vi "Tracking Initialization v2.vi"(5 "Trajectory Cluster":T1, 6 "PID Cluster":T3={"L1 to L4 PID Cluster"={"L1 PID Gains"={"Kp"=0.005, "Kd"=0.5, "Ki"=0.0005}, "L2 PID Gains"={"Kp"=0.01, "Kd"=1.0, "Ki"=0.005}, "L3 PID Gains"={"Kp"=0.05, "Kd"=1.0, "Ki"=0.0005}, "L4 PID Gains"={"Kp"=0.1, "Kd"=0.1, "Ki"=0.0005}}, "Stage PID Cluster"={"Stage Z PID"={"Kp"=0.0005, "Kd"=0.001, "Ki"=0.0}, "Stage Y PID"={"Kp"=0.0003, "Kd"=0.01, "Ki"=0.0}, "Stage X PID"={"Kp"=0.0003, "Kd"=0.01, "Ki"=0.0}}, "OCT Z PID Gains"={"Kp"=0.0003, "Kd"=0.0001, "Ki"=0.01}}, 7 "Offset Home 2 RCM":dbl[](array[numeric])=[0.0, 0.0, 0.0, 0.0], 8 "error in":errorcluster, 10 "Prev Posit Cluster":T4={"Prev L1 to L4 Posit"=[0.0, 0.0, 0.0, 0.0], "Prev Stage Posit"=[6.0, 6.0, 6.0], "Prev OCT Z Posit"=0.0}, 11 "FPGA VI Reference In":refnum<k20>) -> (0 "error out":errorcluster, 2 "Last Posit Cluster":T2={"Last L1 to L4 Posit"=[0.0, 0.0, 0.0, 0.0], "Last Stage Posit"=[6.0, 6.0, 6.0], "Last OCT Z Posit"=0.0}, 3 "FPGA VI Reference Out":refnum<k20>)   [LabVIEW 2016]
uses:
  <vilib>/Platform/TimedLoop/XDataNode/timing_clust.ctl
  <vilib>/Platform/TimedLoop/XDataNode/nitl_modes.ctl
  <vilib>/Platform/TimedLoop/XDataNode/wakeup.ctl
  Global Variables.vi
  <vilib>/platform/TimedLoop/XDataNode/XDataNode.xnode
  <vilib>/Platform/TimedLoop/XDataNode/XDNodeRunTimeDep.lvlib
panel:
  out "In Servo Loop":bool
  out "Indexing Finished?":bool
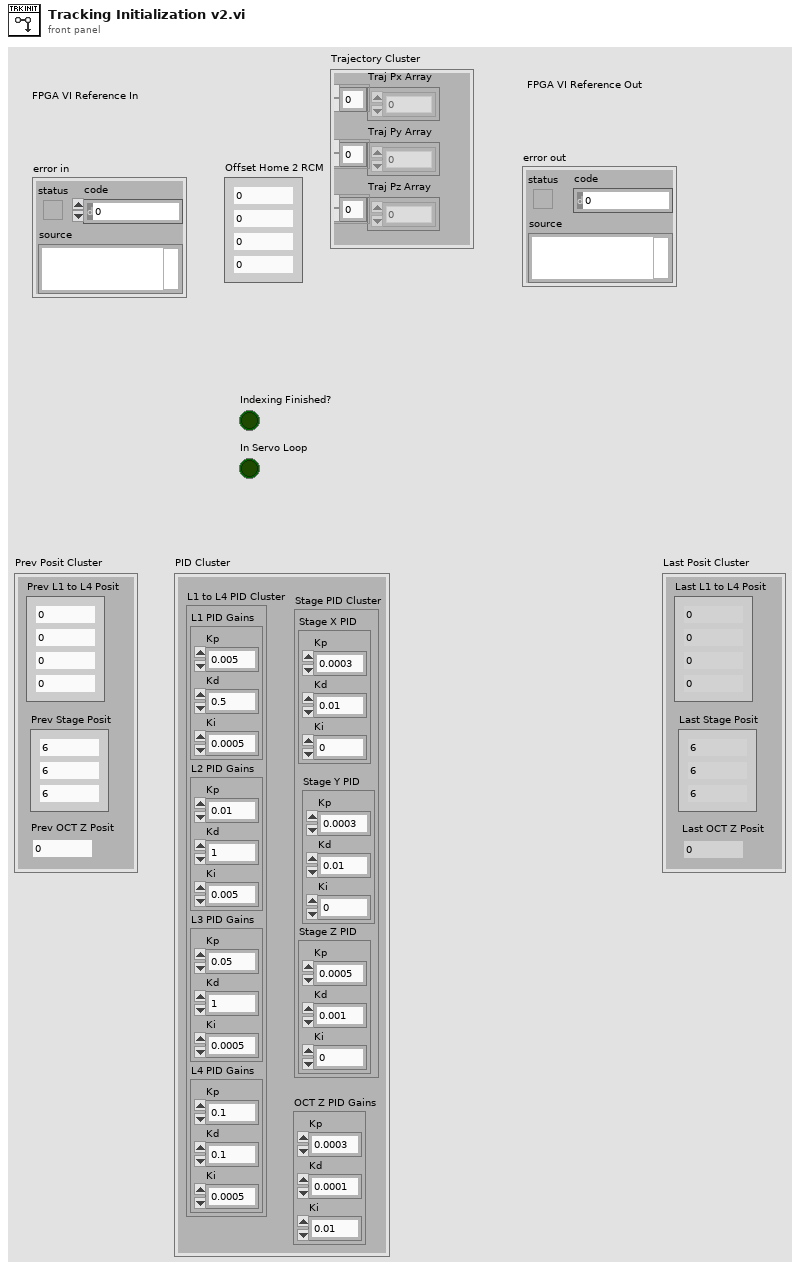
[diagram p1: front panel]
types:
  T1 = cluster{"Traj Px Array":dbl[], "Traj Py Array":dbl[], "Traj Pz Array":dbl[]}
  T2 = cluster{"Last L1 to L4 Posit":dbl[], "Last Stage Posit":dbl[], "Last OCT Z Posit":dbl}
  T3 = cluster{"L1 to L4 PID Cluster":cluster{"L1 PID Gains":cluster{"Kp":dbl, "Kd":dbl, "Ki":dbl}, "L2 PID Gains":cluster{"Kp":dbl, "Kd":dbl, "Ki":dbl}, "L3 PID Gains":cluster{"Kp":dbl, "Kd":dbl, "Ki":dbl}, "L4 PID Gains":cluster{"Kp":dbl, "Kd":dbl, "Ki":dbl}}, "Stage PID Cluster":cluster{"Stage Z PID":cluster{"Kp":dbl, "Kd":dbl, "Ki":dbl}, "Stage Y PID":cluster{"Kp":dbl, "Kd":dbl, "Ki":dbl}, "Stage X PID":cluster{"Kp":dbl, "Kd":dbl, "Ki":dbl}}, "OCT Z PID Gains":cluster{"Kp":dbl, "Kd":dbl, "Ki":dbl}}
  T4 = cluster{"Prev L1 to L4 Posit":dbl[], "Prev Stage Posit":dbl[], "Prev OCT Z Posit":dbl}
  T5 = typedef "XDNodeRunTimeDep.lvlib/timing_clust.ctl" = cluster{"Expected End [f-1]":u64, "Actual End [f-1]":u64, "Finished Late? [f-1]":bool, "Expected End [i-1]":u64, "Actual End [i-1]":u64, "Finished Late? [i-1]":bool, "Expected Start [i]":u64, "Actual Start [i]":u64, "Expected Start [f]":u64, "Actual Start [f]":u64, "Source Name":string, "Structure Name":string, "Period":i64, "Deadline":i64, "Offset":i64, "Start":i64, "Priority":i32, "Timeout":i32, "Mode":T6, "Wakeup Reason":T7, "Error":errorcluster, "Source Type":string, "Secondary Source Type":string, "Global End Time":u64, "Global Start Time":u64, "Frame Duration":u64, "Iteration Duration":u64, "Assigned CPU":i32, "I/O Scan Engine Mode":u32}
  T6 = typedef "XDNodeRunTimeDep.lvlib/nitl_modes.ctl" = enum32{"No Change", "Process missed periods, maintain original phase", "Discard missed periods, maintain original phase", "Process missed periods, ignore original phase", "Discard missed periods, ignore original phase"}
  T7 = typedef "XDNodeRunTimeDep.lvlib/wakeup.ctl" = enum32{"Normal", "Aborted", "Asynchronous wakeup", "Timing source error", "Timed loop error", "Timeout"}
  T8 = cluster{"L1 PID Gains":cluster{"Kp":dbl, "Kd":dbl, "Ki":dbl}, "L2 PID Gains":cluster{"Kp":dbl, "Kd":dbl, "Ki":dbl}, "L3 PID Gains":cluster{"Kp":dbl, "Kd":dbl, "Ki":dbl}, "L4 PID Gains":cluster{"Kp":dbl, "Kd":dbl, "Ki":dbl}}
  T9 = cluster{"Stage Z PID":cluster{"Kp":dbl, "Kd":dbl, "Ki":dbl}, "Stage Y PID":cluster{"Kp":dbl, "Kd":dbl, "Ki":dbl}, "Stage X PID":cluster{"Kp":dbl, "Kd":dbl, "Ki":dbl}}
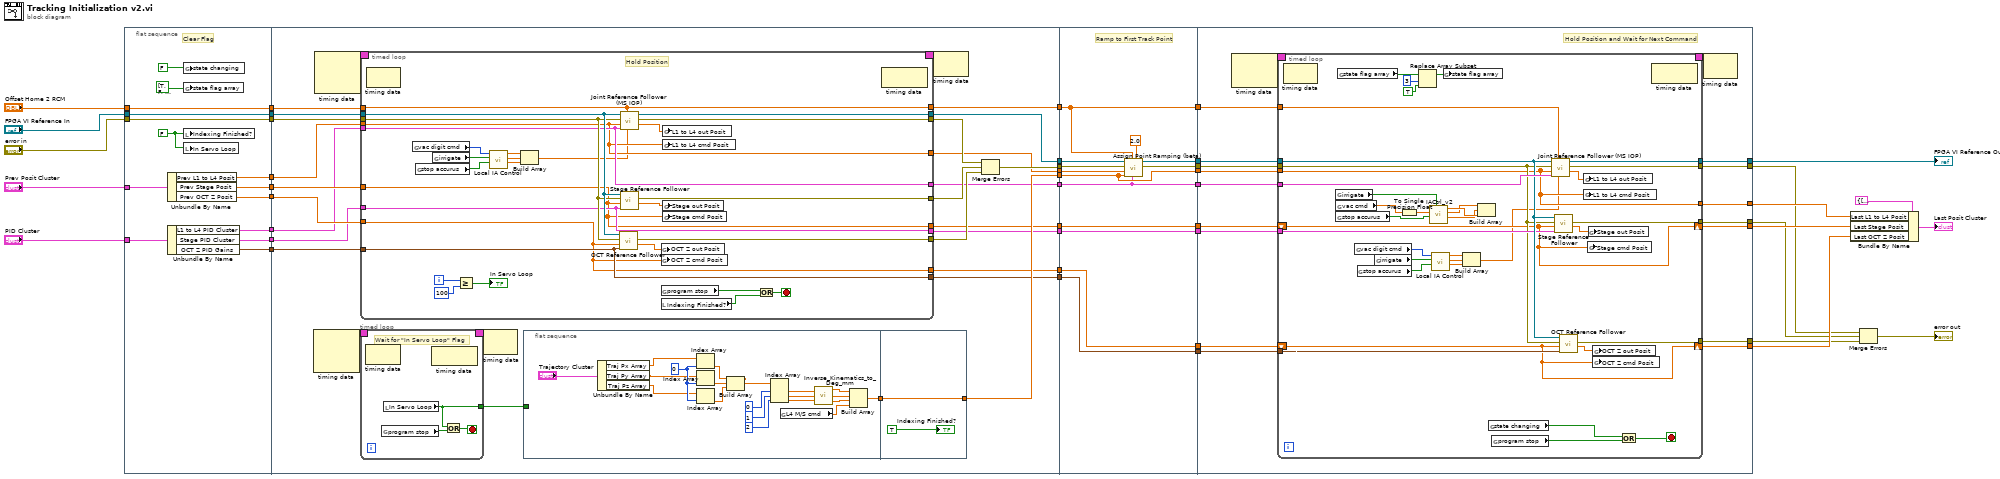
[diagram p0: block diagram]
diagram:
  n1 = flat-sequence {
    tunnel: [w55] -> w21
    tunnel: "FPGA VI Reference In" -> [w55]
    tunnel: "error in" -> [w54]
    tunnel: [w54] -> w19
    tunnel: [w49] -> w17
    tunnel: "PID Cluster" -> [w48]
    tunnel: "Offset Home 2 RCM" -> [w53]
    tunnel: [w53] -> w15
    tunnel: "Prev Posit Cluster" -> [w52]
    tunnel: [w51] -> w12
    tunnel: [w50] -> w10
    tunnel: [w47] -> w8
    tunnel: [w46] -> w7
    tunnel: [w45] -> w6
    tunnel: w21 -> [w82]
    tunnel: [w76] -> w20
    tunnel: w19 -> [w81]
    tunnel: [w72] -> w18
    tunnel: w17 -> [w80]
    tunnel: [w71] -> w16
    tunnel: w15 -> [w83]
    tunnel: [w77] -> w14
    tunnel: [w70] -> w13
    tunnel: w12 -> [w79]
    tunnel: [w68] -> w11
    tunnel: w10 -> [w78]
    tunnel: [w69] -> w9
    tunnel: w8 -> [w67]
    tunnel: w7 -> [w66]
    tunnel: w6 -> [w65]
    tunnel: [w64] -> w5
    tunnel: [w63] -> w3
    tunnel: [w62] -> w1
    tunnel: w20 -> [w160]
    tunnel: w18 -> [w159]
    tunnel: w16 -> [w157]
    tunnel: w14 -> [w154]
    tunnel: w13 -> [w153]
    tunnel: [w156] -> w41
    tunnel: [w153] -> w40
    tunnel: [w155] -> w39
    tunnel: [w154] -> w38
    tunnel: [w150] -> w35
    tunnel: [w148] -> w34
    tunnel: w11 -> [w152]
    tunnel: [w152] -> w22
    tunnel: w9 -> [w149]
    tunnel: w5 -> [w151]
    tunnel: [w151] -> w4
    tunnel: w3 -> [w150]
    tunnel: [w149] -> w2
    tunnel: w1 -> [w148]
    tunnel: [w173] -> w30
    tunnel: [w172] -> w25
    tunnel: w41 -> [w175]
    tunnel: w40 -> [w162]
    tunnel: w39 -> [w176]
    tunnel: w38 -> [w163]
    tunnel: [w171] -> w36
    tunnel: [w170] -> w37
    tunnel: w35 -> [w169]
    tunnel: w34 -> [w168]
    tunnel: [w167] -> w31
    tunnel: [w166] -> w24
    tunnel: [w165] -> w23
    tunnel: w22 -> [w164]
    tunnel: w4 -> [w174]
    tunnel: w2 -> [w161]
    frame #0 {
      w44 = FALSE ("Indexing Finished?")
      # "Clear Flag"
      n2 = Unbundle By Name(w52) -> ("Prev L1 to L4 Posit"=w49:dbl[], "Prev Stage Posit"=w51:dbl[], "Prev OCT Z Posit"=w50:dbl)
      n3 = Unbundle By Name(w48) -> ("L1 to L4 PID Cluster"=w47:T8, "Stage PID Cluster"=w46:T9, "OCT Z PID Gains"=w45:cluster{"Kp":dbl, "Kd":dbl, "Ki":dbl})
      n4 = global write "Global Variables.vi" "state changing"(FALSE ("state changing")) -> ()
      n5 = global write "Global Variables.vi" "state flag array"(bool[] [TRUE, FALSE, FALSE, FALSE, FALSE, FALSE, FALSE, FALSE, FALSE] ("state flag array")) -> ()
      n6 = local write "Indexing Finished?"(w44) -> ()
      n7 = local write "In Servo Loop"(w44) -> ()
    }
    frame #1 {
      n8 = node-c288() -> (w61:T5)  [unwired: 3 in]
      n9 = node-c288() -> (w85:T5)  [unwired: 3 in]
      n10 = timed-loop {
        timing: w61 -> [_]
        timing-out: [_] -> w60
        tunnel: [w108] -> w59
        stop <- w110 stop-if-true
        # "Wait for \"In Servo Loop\" Flag"
        n11 = node-c288() -> ()  [unwired: 1 in, 1 out]
        n12 = global read "Global Variables.vi" "program stop"() -> (w109:bool)
        n13 = local read "In Servo Loop"() -> (w108:bool)
        n14 = node-c288() -> ()  [unwired: 1 in, 1 out]
        n15 = Or(x=w108, y=w109) -> (x .or. y?=w110:bool)
      }
      n16 = timed-loop {
        timing: w85 -> [_]
        timing-out: [_] -> w84
        tunnel: w83 -> [w141]
        tunnel: w82 -> [w143]
        tunnel: w81 -> [w142]
        tunnel: w80 -> [w124]
        tunnel: w79 -> [w123]
        tunnel: w78 -> [w122]
        tunnel: [w141] -> w77
        tunnel: [w140] -> w76
        tunnel: [w139] -> w75
        tunnel: [w138] -> w74
        tunnel: [w137] -> w73
        tunnel: [w124] -> w71
        tunnel: [w123] -> w68
        tunnel: [w122] -> w69
        tunnel: w67 -> [w130]
        tunnel: w66 -> [w129]
        tunnel: w65 -> [w128]
        tunnel: [w130] -> w64
        tunnel: [w129] -> w63
        tunnel: [w128] -> w62
        i -> [w127]
        stop <- w132 stop-if-true
        # "Hold Position"
        n17 = node-c288() -> ()  [unwired: 1 in, 1 out]
        n18 = global read "Global Variables.vi" "vac digit cmd"() -> (w120:i8)
        n19 = global read "Global Variables.vi" "stop accurus"() -> (w119:bool)
        n20 = global read "Global Variables.vi" "irrigate"() -> (w121:bool)
        n21 = Greater Or Equal?(x=w127, y=100) -> (x >= y?=→"In Servo Loop":bool)
        n22 = call "Local IA Control.vi"("E-Stop Vacuum"=w119, "Irrigate?"=w121, "8bit integer"=w120) -> ("Accurus Engaged Vout"=w116:dbl, "Accurus ChB Vout"=w117:dbl, "Accurus ChA Vout"=w118:dbl)  [unwired: 6 in]
        n23 = Build Array(w118, w117, w116) -> (w115:dbl[])
        n24 = call "OCT Reference Follower.vi"("OCT Z PID Gains"=w128, "OCT  Z cmd Posit [mm]"=w122, "error in"=w142, "FPGA VI Reference In"=w143) -> ("OCT  Z out Posit [mm]"=w134:dbl, "error out"=w137:errorcluster)  [unwired: 5 in, 1 out]
        n25 = call "Joint Reference Follower (MS IOP).vi"("Acc Ctrl Array"=w115, "Offset Home2RCM [deg/mm]"=w141, "PID Ctrl Cluster"=w130, "Ref Array [deg/mm]"=w124, "error in"=w142, "FPGA VI Reference In"=w143) -> ("Output Posit Array [deg/mm]"=w136:dbl[], "error out"=w139:errorcluster, "FPGA VI Reference Out"=w140:refnum<k20>)  [unwired: 3 in]
        n26 = call "Stage Reference Follower.vi"("Stage PID Cluster"=w129, "Stage cmd Posit [mm]"=w123, "error in"=w142, "FPGA VI Reference In"=w143) -> ("Stage out Posit [mm]"=w135:dbl[], "error out"=w138:errorcluster)  [unwired: 5 in, 1 out]
        n27 = global write "Global Variables.vi" "OCT Z out Posit"(w134) -> ()
        n28 = global write "Global Variables.vi" "OCT Z cmd Posit"(w122) -> ()
        n29 = global read "Global Variables.vi" "program stop"() -> (w133:bool)
        n30 = local read "Indexing Finished?"() -> (w131:bool)
        n31 = global write "Global Variables.vi" "L1 to L4 out Posit"(w136) -> ()
        n32 = global write "Global Variables.vi" "L1 to L4 cmd Posit"(w124) -> ()
        n33 = global write "Global Variables.vi" "Stage out Posit"(w135) -> ()
        n34 = global write "Global Variables.vi" "Stage cmd Posit"(w123) -> ()
        n35 = Or(x=w133, y=w131) -> (x .or. y?=w132:bool)
        n36 = node-c288() -> ()  [unwired: 1 in, 1 out]
      }
      n37 = node-c288(w60) -> ()  [unwired: 1 out]
      n38 = flat-sequence {
        tunnel: w59 -> [_]
        tunnel: [w87] -> w58
        tunnel: [w106] -> w70
        tunnel: w58 -> [w106]
        frame #0 {
          w92 = 0 ("index")
          n39 = Unbundle By Name("Trajectory Cluster") -> ("Traj Px Array"=w88:dbl[], "Traj Py Array"=w90:dbl[], "Traj Pz Array"=w89:dbl[])
          n40 = Index Array(array=w88, index=w92) -> (element=w104:dbl)
          n41 = Index Array(array=w90, index=w92) -> (element=w103:dbl)
          n42 = Index Array(array=w89, index=w92) -> (element=w102:dbl)
          n43 = Build Array(w104, w103, w102) -> (w91:dbl[])
          n44 = Index Array(array=w91, index #1=0 ("index"), index #2=1 ("index"), index #3=2 ("index")) -> (element #1=w97:dbl, element #2=w95:dbl, element #3=w96:dbl)
          n45 = global read "Global Variables.vi" "L4 M/S cmd"() -> (w86:dbl)
          n46 = call "Inverse_Kinematics_to_Deg_mm.vi"("pz"=w96, "py"=w95, "px"=w97) -> ("L3 [mm]"=w100:dbl, "L2 [deg]"=w99:dbl, "L1 [deg]"=w98:dbl)
          n47 = Build Array(w98, w99, w100, w86) -> (w87:dbl[])
        }
        frame #1 {
          "Indexing Finished?" <- TRUE ("Indexing Finished?")
        }
      }
      n48 = node-c288(w84) -> ()  [unwired: 1 out]
      n49 = Merge Errors(w75, w74, w73) -> (w72:errorcluster)
    }
    frame #2 {
      # "Ramp to First Track Point"
      n50 = call "Assign Point Ramping (beta).vi"("Ramp Time [sec]"=2.0, "L1 to L4 PID Cluster"=w151, "Offset Home2RCM"=w154, "Destination Posit Array [mm]"=w153, "Previous Posit Array"=w157, "error in"=w159, "FPGA VI Reference In"=w160) -> ("error out"=w156:errorcluster, "FPGA VI Reference Out"=w155:refnum<k20>)  [unwired: 2 in, 1 out]
    }
    frame #3 {
      # "Hold Position and Wait for Next Command"
      n51 = node-c288() -> (w178:T5)  [unwired: 2 in]
      n52 = timed-loop {
        timing: w178 -> [_]
        timing-out: [_] -> w177
        tunnel: w176 -> [w205]
        tunnel: w175 -> [w198]
        tunnel: w163 -> [w210]
        tunnel: w162 -> [w195]
        tunnel: w174 -> [w209]
        tunnel: [w208] -> w173
        tunnel: [w207] -> w172
        tunnel: [w195] -> w171
        tunnel: w169 -> [w202]
        tunnel: w168 -> [w201]
        tunnel: [w197] -> w166
        tunnel: [w196] -> w165
        shift-right: [w194] -> w170
        shift-left: w164 -> [w194]
        shift-right: [w193] -> w167
        shift-left: w161 -> [w193]
        stop <- w199 stop-if-true
        # "Hold Position if not Engaged"
        n53 = node-c288() -> ()  [unwired: 1 in, 1 out]
        n54 = global read "Global Variables.vi" "irrigate"() -> (w191:bool)
        n55 = global read "Global Variables.vi" "vac cmd"() -> (w188:sgl)
        n56 = global read "Global Variables.vi" "stop accurus"() -> (w187:bool)
        n57 = global read "Global Variables.vi" "state flag array"() -> (w214:bool[])
        n58 = global read "Global Variables.vi" "vac digit cmd"() -> (w184:i8)
        n59 = global read "Global Variables.vi" "stop accurus"() -> (w183:bool)
        n60 = global read "Global Variables.vi" "irrigate"() -> (w185:bool)
        n61 = To Single Precision Float(number=w188) -> (single precision float=w189:sgl)
        n62 = Replace Array Subset(array=w214, new element=TRUE ("new element/subarray"), index=3) -> (w213:bool[])
        n63 = call "IACtrl_v2.vi"("Irrigate?"=w191, "E-Stop Vacuum"=w187, "Vacuum Force [mmHg]"=w189) -> ("Accurus ChB Vout"=w186:dbl, "Accurus ChA Vout"=w190:dbl, "Accurus Engaged Vout"=w192:dbl)  [unwired: 5 in, 1 out]
        n64 = call "Local IA Control.vi"("E-Stop Vacuum"=w183, "Irrigate?"=w185, "8bit integer"=w184) -> ("Accurus Engaged Vout"=w180:dbl, "Accurus ChB Vout"=w181:dbl, "Accurus ChA Vout"=w182:dbl)  [unwired: 6 in]
        n65 = global write "Global Variables.vi" "state flag array"(w213) -> ()
        n66 = Build Array(w182, w181, w180) -> (w179:dbl[])
        n67 = Build Array(w190, w186, w192) -> ()  [unwired: 1 out]
        n68 = global read "Global Variables.vi" "state changing"() -> (w215:bool)
        n69 = global read "Global Variables.vi" "program stop"() -> (w204:bool)
        n70 = call "Joint Reference Follower (MS IOP).vi"("Acc Ctrl Array"=w179, "Offset Home2RCM [deg/mm]"=w210, "PID Ctrl Cluster"=w209, "Ref Array [deg/mm]"=w195, "error in"=w198, "FPGA VI Reference In"=w205) -> ("Output Posit Array [deg/mm]"=w203:dbl[], "error out"=w207:errorcluster, "FPGA VI Reference Out"=w208:refnum<k20>)  [unwired: 3 in]
        n71 = call "Stage Reference Follower.vi"("Stage PID Cluster"=w202, "Stage cmd Posit [mm]"=w194, "error in"=w198, "FPGA VI Reference In"=w205) -> ("Stage out Posit [mm]"=w206:dbl[], "error out"=w197:errorcluster)  [unwired: 5 in, 1 out]
        n72 = call "OCT Reference Follower.vi"("OCT Z PID Gains"=w201, "OCT  Z cmd Posit [mm]"=w193, "error in"=w198, "FPGA VI Reference In"=w205) -> ("OCT  Z out Posit [mm]"=w200:dbl, "error out"=w196:errorcluster)  [unwired: 5 in, 1 out]
        n73 = global write "Global Variables.vi" "L1 to L4 out Posit"(w203) -> ()
        n74 = global write "Global Variables.vi" "L1 to L4 cmd Posit"(w195) -> ()
        n75 = global write "Global Variables.vi" "Stage cmd Posit"(w194) -> ()
        n76 = global write "Global Variables.vi" "Stage out Posit"(w206) -> ()
        n77 = global write "Global Variables.vi" "OCT Z out Posit"(w200) -> ()
        n78 = global write "Global Variables.vi" "OCT Z cmd Posit"(w193) -> ()
        n79 = Or(x=w215, y=w204) -> (x .or. y?=w199:bool)
        n80 = node-c288() -> ()  [unwired: 1 in, 1 out]
      }
      n81 = node-c288(w177) -> ()  [unwired: 1 out]
    }
  }
  n82 = Bundle By Name(cluster=T2 {"Last L1 to L4 Posit"=[0.0, 0.0, 0.0, 0.0], "Last Stage Posit"=[6.0, 6.0, 6.0], "Last OCT Z Posit"=0.0} ("Last Posit Cluster 2"), "Last L1 to L4 Posit"=w36, "Last Stage Posit"=w37, "Last OCT Z Posit"=w31) -> (→"Last Posit Cluster":T2)
  n83 = Merge Errors(w25, w24, w23) -> (→"error out":errorcluster)
  "FPGA VI Reference Out" <- w30
